vi "Update Chart Title.vi"(8 "error in (no error)":errorcluster, 10 "Chart Title":string, 11 "Boolean in":refnum<vi>) -> (0 "error out":errorcluster)   [LabVIEW 2014, in "Chart Module.lvlib"]
uses:
  Chart Module.lvlib
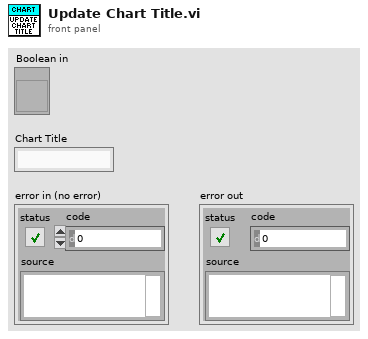
[diagram p1: front panel]
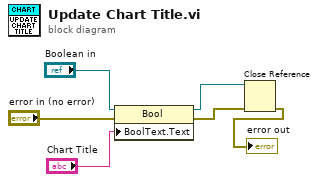
[diagram p0: block diagram]
diagram:
  n1 = property on="Property Node" class="Bool"(reference="Boolean in", error in="error in (no error)", "BoolText.Text"="Chart Title") -> (reference out=w3:refnum<vi>, error out=w1:errorcluster)
  n2 = Close Reference(reference=w3, error in (no error)=w1) -> (error out=→"error out":errorcluster)
